vi "commandQueues.vi"(8 "ErrorIn":errorcluster, 9 "CommandIn":T1, 10 "CommandQueuesAction":T3=enum."Get", 11 "Threads":T2[](array[typedef])) -> (0 "ErrorOut":errorcluster, 1 "CommandOut":T1)   [LabVIEW 2019]
uses:
  CommandQueuesAction.ctl
  Thread.ctl
  Command.ctl
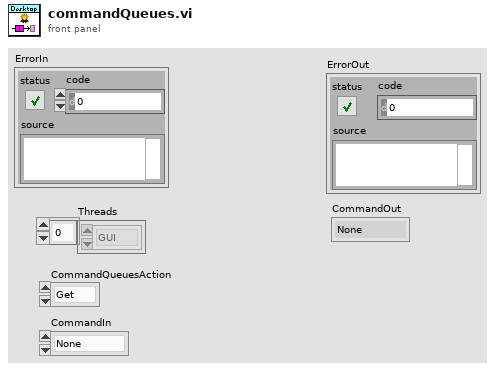
[diagram p1: front panel]
types:
  T1 = typedef "Command.ctl" = enum16{"None", "Connect", "Start", "Stop", "RestartAnalyzer", "Exit", "OpenDataFile", "CanBegin"}
  T2 = typedef "Thread.ctl" = enum16{"GUI", "communicateWithAnalyzer", "saveDataToTDMS"}
  T3 = typedef "CommandQueuesAction.ctl" = enum16{"Initialize", "Set", "Get", "ReleaseAll"}
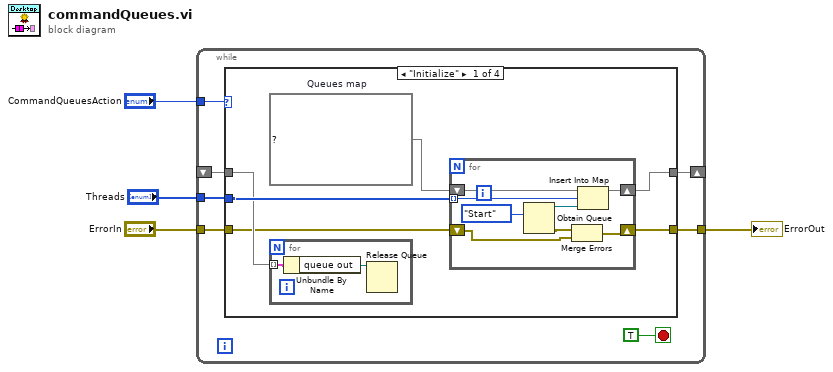
[diagram p0: block diagram]
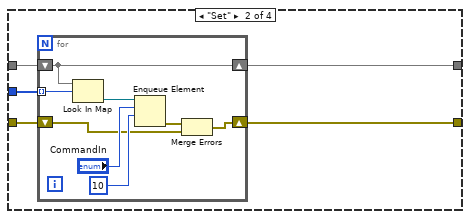
[diagram p2: hidden frame]
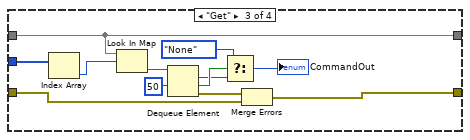
[diagram p3: hidden frame]
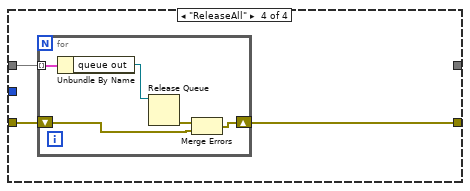
[diagram p4: hidden frame]
diagram:
  n1 = while {
    tunnel: "CommandQueuesAction" -> [w11]
    tunnel: "Threads" -> [w10]
    shift-right: [w8] -> _
    shift-left: _ -> [w6]
    tunnel: "ErrorIn" -> [w9]
    tunnel: [w5] -> w2
    stop <- TRUE stop-if-true
    n2 = case shown="\"Initialize\"" w11 {
      tunnel: w10 -> [w17 w31 w48 _]
      tunnel: w9 -> [w12 w28 w45 w54]
      tunnel: [w16 w29 w51 _] -> w8
      tunnel: w6 -> [w13 w32 w51 w55]
      tunnel: [w14 w30 w46 w53] -> w5
      frame "Initialize" {
        w15 = map{T2, refnum<queue>} {}  # Queues map
        n3 = for {
          tunnel: w13 -> [w19] mode=indexing
          n4 = Unbundle By Name(w19) -> ("queue out"=w18:refnum<queue>)
          n5 = Release Queue(queue=w18) -> ()  [unwired: 2 in, 3 out]
        }
        n6 = for {
          tunnel: w17 -> [w26] mode=indexing
          shift-right: [w21] -> w14
          shift-left: w12 -> [w20]
          shift-right: [w25] -> w16
          shift-left: w15 -> [w27]
          n7 = Obtain Queue(element data type=Command."Start" ("Command")) -> (queue out=w23:refnum<queue>, error out=w22:errorcluster)  [unwired: 4 in, 1 out]
          n8 = Merge Errors(w22, w20) -> (w21:errorcluster)
          n9 = Insert Into Map(map in=w27, key=w26, value=w23) -> (map out=w25:map{T2, refnum<queue>})  [unwired: 2 out]
        }
      }
      frame "Set" {
        n10 = for {
          tunnel: w31 -> [w40] mode=indexing
          shift-right: [w34] -> w30
          shift-left: w28 -> [w33]
          shift-right: [w35] -> w29
          shift-left: w32 -> [w35]
          n11 = Look In Map(map=w35, key=w40) -> (value=w39:refnum<queue>)  [unwired: 1 in, 1 out]
          n12 = Enqueue Element(queue=w39, element="CommandIn", timeout in ms (-1)=10) -> (error out=w36:errorcluster)  [unwired: 1 in, 2 out]
          n13 = Merge Errors(w36, w33) -> (w34:errorcluster)
        }
      }
      frame "Get" {
        n14 = Index Array(array=w48) -> (element=w47:T2)  [unwired: 1 in]
        n15 = Look In Map(map=w51, key=w47) -> (value=w50:refnum<queue>)  [unwired: 1 in, 1 out]
        n16 = Dequeue Element(queue=w50, timeout in ms (-1)=50) -> (element=w43:T1, timed out?=w44:bool, error out=w52:errorcluster)  [unwired: 1 in, 1 out]
        n17 = Select(t=Command."None", s=w44, f=w43) -> (s? t:f=→"CommandOut":T1)
        n18 = Merge Errors(w52, w45) -> (w46:errorcluster)
      }
      frame "ReleaseAll" {
        n19 = for {
          tunnel: w55 -> [w60] mode=indexing
          shift-right: [w57] -> w53
          shift-left: w54 -> [w56]
          n20 = Unbundle By Name(w60) -> ("queue out"=w59:refnum<queue>)
          n21 = Release Queue(queue=w59) -> (error out=w58:errorcluster)  [unwired: 2 in, 2 out]
          n22 = Merge Errors(w58, w56) -> (w57:errorcluster)
        }
      }
    }
  }
  "ErrorOut" <- w2
